vi "Clear Data.vi"(8 "error in (no error)":errorcluster, 10 "AcqID":i32, 11 "Automation Refnum in":refnum<k7>) -> (0 "error out":errorcluster)   [LabVIEW 2014]
uses:
  Exec Command.ctl
panel:
  out "Failed":bool
  # "LICENSED MATERIALS – PROPERTY OF IBM\nCopyright IBM Corp. 2016,\nALL RIGHTS RESERVED"
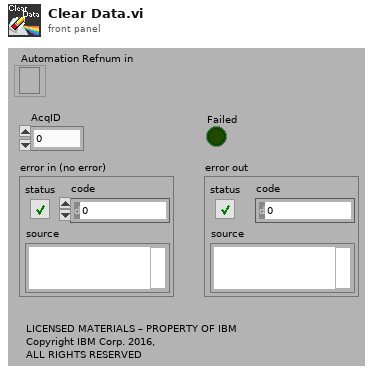
[diagram p1: front panel]
types:
  T1 = typedef "Exec Command.ctl" = u16
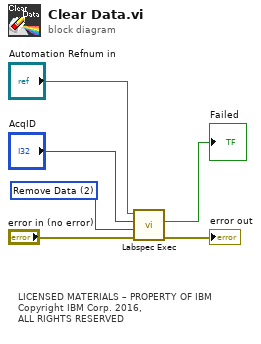
[diagram p0: block diagram]
diagram:
  w1 = T1 2 items=["Show data", "Hide data", "Remove Data", "Clone Data", "Show Style", "Show Mode", "Show Axis", "Hide all"] ("Command")
  # "LICENSED MATERIALS – PROPERTY OF IBM\nCopyright IBM Corp. 2016,\nALL RIGHTS RESERVED"
  n1 = call "Labspec Exec.vi"("error in"="error in (no error)", "Command"=w1, "Data ID"="AcqID", "Automation Refnum In"="Automation Refnum in") -> ("error out"=→"error out":errorcluster, "Failed"=→"Failed":bool)  [unwired: 4 in, 2 out]
